vi "Generate File Header.vi"() -> ()   [LabVIEW 2012]
uses:
  Header Data.ctl
panel:
  out "文件头":string
  in  "文件头数据":T1={"操作员姓名"="Fred", "UUT序列号"="A001", "测试名称"="测试系统"}
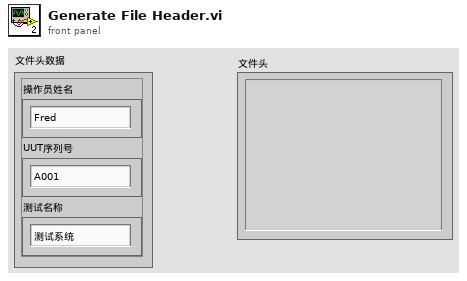
[diagram p1: front panel]
types:
  T1 = typedef "Header Data.ctl" = cluster{"操作员姓名":string, "UUT序列号":string, "测试名称":string}
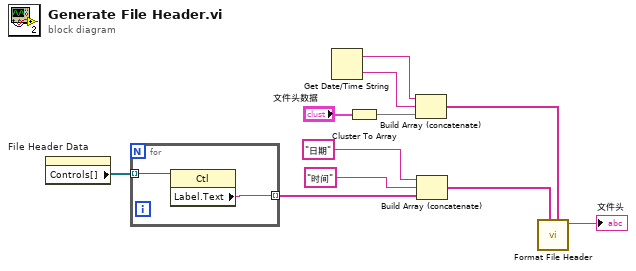
[diagram p0: block diagram]
diagram:
  n1 = property on="File Header Data" class="Clust (严格)"() -> ("Controls[]"=w10:refnum<vi>[])  [unwired: 2 in, 2 out]
  n2 = for {
    tunnel: w10 -> [w13] mode=indexing
    tunnel: [w12] -> w8 mode=indexing
    n3 = property on="属性节点" class="Ctl"(reference=w13) -> ("Label.Text"=w12:string)  [unwired: 1 in, 2 out]
  }
  n4 = Get Date/Time String ("获取日期/时间字符串")() -> (date string=w4:string, time string=w5:string)  [unwired: 3 in]
  n5 = Cluster To Array ("簇至数组转换")(cluster="文件头数据") -> (array=w9:string[])
  n6 = Build Array (concatenate) ("创建数组")(w4, w5, w9) -> (w2:string[])
  n7 = Build Array (concatenate) ("创建数组")("日期", "时间", w8) -> (w3:string[])
  n8 = call "Format File Header.vi"("头信息数据（空）"=w2, "头信息标题（空）"=w3) -> ("文件头"=→"文件头":string)  [unwired: 8 in, 1 out]
